vi "Set Scroll.vi"(8 "error in (no error)":errorcluster, 10 "Position":T1, 11 "2DArrayManager in":refnum<class "2DArrayManager.lvclass">) -> (0 "error out":errorcluster, 3 "2DArrayManager out":refnum<class "2DArrayManager.lvclass">)   [LabVIEW 2020, in "OOPanel.lvlib" / "2DArrayManager.lvclass"]
uses:
  2DArrayManager.lvclass
  2D Position.ctl
  OOPanel.lvlib
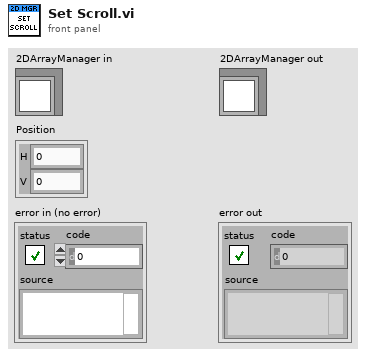
[diagram p1: front panel]
types:
  T1 = typedef "OOPanel.lvlib/2D Position.ctl" = cluster{"H":i32, "V":i32}
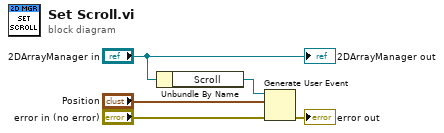
[diagram p0: block diagram]
diagram:
  n1 = Unbundle By Name("2DArrayManager in") -> ("Scroll"=w4:refnum<user-event>)
  n2 = Generate User Event(user event=w4, event data cluster="Position", error in="error in (no error)") -> (error out=→"error out":errorcluster)  [unwired: 1 in, 1 out]
  "2DArrayManager out" <- "2DArrayManager in"
